vi "all_elements_present.vi"(8 "error in (no error)":errorcluster, 11 "multicolumn list box":refnum<vi>) -> (0 "error out":errorcluster, 3 "all elements are present":bool)   [LabVIEW 2010]
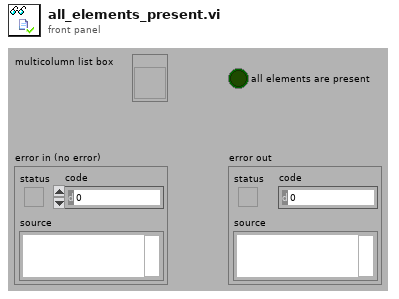
[diagram p1: front panel]
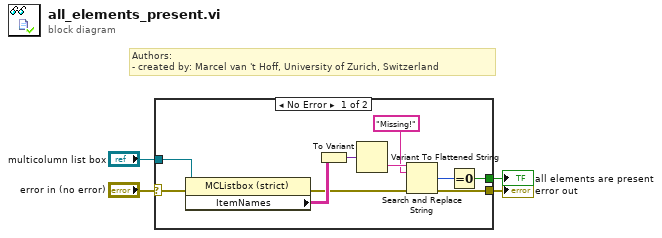
[diagram p0: block diagram]
diagram:
  # "Authors: \n- created by: Marcel van 't Hoff, University of Zurich, Switzerland"
  n1 = case shown="No Error" "error in (no error)" {
    selector: "error in (no error)" -> [w13 w15]
    tunnel: "multicolumn list box" -> [w14 _]
    tunnel: [w7 _] -> w2
    tunnel: [w5 w15] -> w1
    frame No Error {
      n2 = property class="MCListbox (strict)"(reference=w14, error in=w13) -> (error out=w6:errorcluster, "ItemNames"=w12:string[][])  [unwired: 1 out]
      n3 = To Variant(anything=w12) -> (Variant=w11:variant)
      n4 = Variant To Flattened String(Variant=w11) -> (data string=w10:string)  [unwired: 1 out]
      n5 = Search and Replace String(input string=w10, search string="Missing!" ("f"), error in=w6) -> (number of replacements=w8:i32, error out=w5:errorcluster)  [unwired: 5 in, 2 out]
      n6 = Equal To 0?(x=w8) -> (x = 0?=w7:bool)
    }
    frame Error {
    }
  }
  "all elements are present" <- w2
  "error out" <- w1
